vi "writeToSerialAcq.vi"(0 "Cmmd":string="*idn?", 1 "input COM Port":refnum<visa-resource-name>="COM10") -> ()   [LabVIEW 2015]
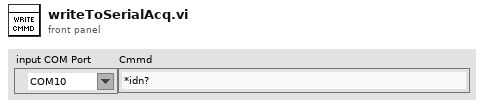
[diagram p1: front panel]
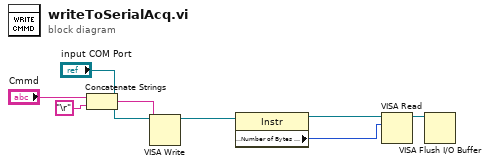
[diagram p0: block diagram]
diagram:
  n1 = Concatenate Strings("Cmmd", "\r") -> (w8:string)
  n2 = VISA Write(VISA resource name="input COM Port", write buffer=w8) -> (VISA resource name out=w3:refnum<visa-resource-name>)  [unwired: 1 in, 2 out]
  n3 = property class="Instr"(reference=w3) -> (reference out=w2:refnum<visa-resource-name>, "Serial Settings:Number of Bytes at Serial Port"=w4:u32)  [unwired: 1 in, 1 out]
  n4 = VISA Read(VISA resource name=w2, byte count=w4) -> (VISA resource name out=w1:refnum<visa-resource-name>)  [unwired: 1 in, 3 out]
  n5 = VISA Flush I/O Buffer(VISA resource name=w1) -> ()  [unwired: 2 in, 2 out]
